vi "comparison operator.vi"() -> ()   [LabVIEW 2017]
panel:
  out "x > y?":bool
  in  "y":dbl
  in  "x":dbl
  out "x != y?":bool
  out "x = y?":bool
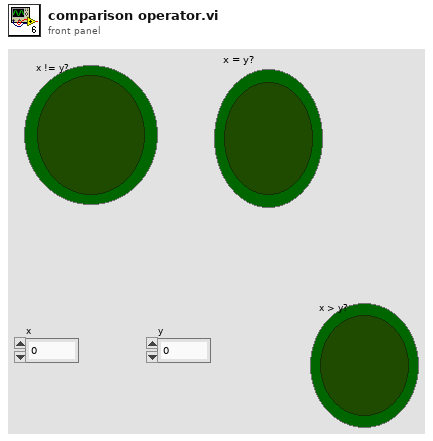
[diagram p1: front panel]
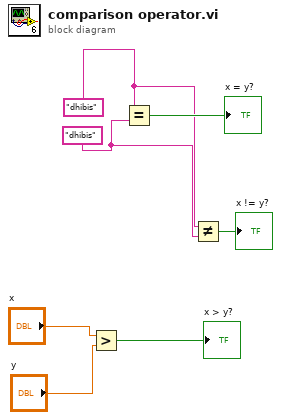
[diagram p0: block diagram]
diagram:
  w5 = "dhibis"
  w6 = "dhibis" ("x")
  n1 = Greater?(x="x", y="y") -> (0:→"x > y?":bool)
  n2 = Equal?(x=w6, y=w5) -> (x = y?=→"x = y?":bool)
  n3 = Not Equal?(x=w6, y=w5) -> (x != y?=→"x != y?":bool)
